vi "AutonTxtFile.vi"(0 "enum":T1=enum."Initialize", 1 "dataName":string, 2 "mode":T2(ring), 3 "reset?":bool, 5 "integer":i32, 7 "float":dbl format="%#_13g", 9 "boolean":bool, 11 "string":string, 12 "newLine?":bool, 13 "writeToFile?":bool, 14 "doubleSpace?":bool) -> (4 "flowControl":string, 15 "flowControl2":i32)   [LabVIEW 2017]
uses:
  Auton.ctl
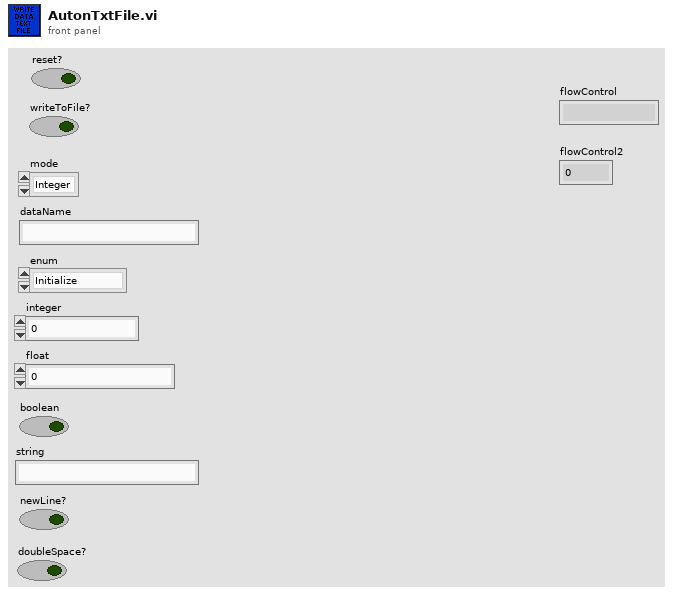
[diagram p1: front panel]
types:
  T1 = typedef "Auton.ctl" = enum16{"VisionTarget", "Wait", "Initialize", "Stop", "Reset", "StraightForward", "StraightBack", "SolenoidControl", "SharpLeftCurve", "SharpRightCurve", "GradLeftCurve", "GradRightCurve", "TurnLeft90", "TurnRight90", "TurnLeft60", "TurnRight60", "TurnLeft45", "TurnRight45", "Shoot", "SpinUp", "GearApproach", "ShortShoot", "SlowForward", "TimeForward", "Pause", "HopperDrive"}
  T2 = enum16{"Integer", "Float", "Boolean", "Enum", "String"}
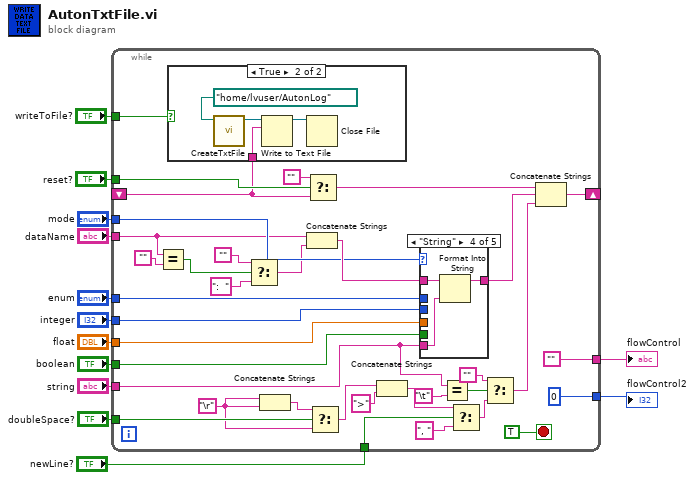
[diagram p0: block diagram]
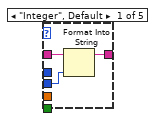
[diagram p3: hidden frame]
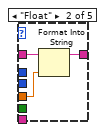
[diagram p4: hidden frame]
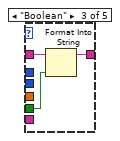
[diagram p5: hidden frame]
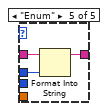
[diagram p6: hidden frame]
diagram:
  n1 = while {
    tunnel: "mode" -> [w35]
    tunnel: "dataName" -> [w24]
    tunnel: "integer" -> [w49]
    tunnel: "float" -> [w48]
    tunnel: "enum" -> [w47]
    tunnel: "boolean" -> [w46]
    tunnel: "writeToFile?" -> [w45]
    tunnel: "newLine?" -> [w29]
    tunnel: "string" -> [w18]
    tunnel: "doubleSpace?" -> [w42]
    shift-right: [w38] -> _
    shift-left: _ -> [w14]
    tunnel: "reset?" -> [w34]
    tunnel: [""] -> w3
    tunnel: [0] -> w2
    stop <- TRUE stop-if-true
    w40 = "\r"
    n2 = Equal?(x=w24, y="") -> (x = y?=w15:bool)
    n3 = case shown="True" w45 {
      tunnel: w14 -> [_ w51]
      frame False {
      }
      frame True {
        n4 = call "CreateTxtFile.vi"("pathIn"=path "/home/lvuser/AutonLog") -> ("refnumOut"=w52:refnum<file>)  [unwired: 10 in]
        n5 = Write to Text File(file (use dialog)=w52, text=w51) -> (refnum out=w53:refnum<file>)  [unwired: 2 in, 2 out]
        n6 = Close File(refnum=w53) -> ()  [unwired: 1 in, 2 out]
      }
    }
    n7 = Select(t="", s=w15, f=":  ") -> (s? t:f=w30:string)
    n8 = Concatenate Strings(w40, w40) -> (w41:string)
    n9 = Concatenate Strings(w24, w30) -> (w43:string)
    n10 = Select(t="", s=w34, f=w14) -> (s? t:f=w36:string)
    n11 = Select(t=w41, s=w42, f=w40) -> (s? t:f=w26:string)
    n12 = Concatenate Strings(w26, ">" ("string")) -> (w21:string)
    n13 = case shown="\"String\"" w35 {
      tunnel: w49 -> [w55 _ _ _ _]
      tunnel: w48 -> [_ w58 _ _ _]
      tunnel: w47 -> [_ _ _ _ w68]
      tunnel: w46 -> [_ _ w61 _ _]
      tunnel: w43 -> [w56 w59 w62 w65 w67]
      tunnel: [w54 w57 w60 w63 w66] -> w39
      tunnel: w18 -> [_ _ _ w64 _]
      frame "Integer", Default {
        n14 = Format Into String(initial string=w56, w55) -> (resulting string=w54:string)  [unwired: 2 in, 1 out]
      }
      frame "Float" {
        n15 = Format Into String(initial string=w59, w58) -> (resulting string=w57:string)  [unwired: 2 in, 1 out]
      }
      frame "Boolean" {
        n16 = Format Into String(initial string=w62, w61) -> (resulting string=w60:string)  [unwired: 2 in, 1 out]
      }
      frame "String" {
        n17 = Format Into String(initial string=w65, w64) -> (resulting string=w63:string)  [unwired: 2 in, 1 out]
      }
      frame "Enum" {
        n18 = Format Into String(initial string=w67, w68) -> (resulting string=w66:string)  [unwired: 2 in, 1 out]
      }
    }
    n19 = Equal?(x=w18, y="\t") -> (x = y?=w20:bool)
    n20 = Select(t=w21, s=w29, f=", ") -> (s? t:f=w23:string)
    n21 = Select(t="", s=w20, f=w23) -> (s? t:f=w17:string)
    n22 = Concatenate Strings(w36, w39, w17) -> (w38:string)
  }
  "flowControl" <- w3
  "flowControl2" <- w2
